vi "new_thread.vi"(6 "done?":bool, 8 "error in (no error)":errorcluster, 11 "Lua Thread in":refnum<class "Lua Thread.lvclass">) -> (0 "error out":errorcluster, 3 "Lua Thread out":refnum<class "Lua Thread.lvclass">)   [LabVIEW 2020, in "Lua for LabVIEW.lvlib" / "Lua Thread.lvclass"]
uses:
  Lua Thread.lvclass
  Lua Thread.lvclass/Lua Thread.ctl
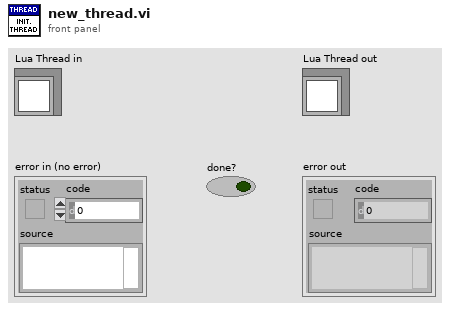
[diagram p1: front panel]
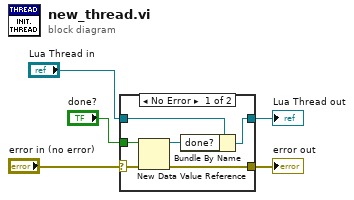
[diagram p0: block diagram]
diagram:
  n1 = case shown="No Error" "error in (no error)" {
    selector: "error in (no error)" -> [w7 w13]
    tunnel: [w8 w13] -> w4
    tunnel: [w10 w12] -> w2
    tunnel: "Lua Thread in" -> [w11 w12]
    tunnel: "done?" -> [w6 _]
    frame No Error {
      n2 = New Data Value Reference(data value=w6, error in=w7) -> (data value reference=w9:refnum<data-value>, error out=w8:errorcluster)
      n3 = Bundle By Name(cluster=w11, "done?"=w9) -> (w10:refnum<class "Lua Thread.lvclass">)
    }
    frame Error {
    }
  }
  "error out" <- w4
  "Lua Thread out" <- w2
